vi "Image & ROI Update(SubVI).vi"(5 "Nr of Objects":dbl, 8 "error in (no error)":errorcluster, 9 "Numeric":dbl=50.0 format="%#_13g", 10 "Optical Flow Previous Image":T1, 11 "Refnum in":T1) -> (0 "error out":errorcluster, 1 "Rectangle":cluster{dbl, dbl, dbl, dbl, dbl}, 2 "ROI Descriptor":T2 {"Contours"."Type" items=["No Selection", "Point", "Line", "Rectangle", "Oval", "Polygon", "Freehand Region", "Annulus", "Unused2", "Unused3", "Broken Line", "Freehand Line", "Rotated Rectangle"]}, 3 "Refnum out":T1)   [LabVIEW 2014]
uses:
  <vilib>/vision/Image Controls.llb/IMAQ Image.ctl
  Global.vi
  <vilib>/vision/NI_Vision_Development_Module.lvlib
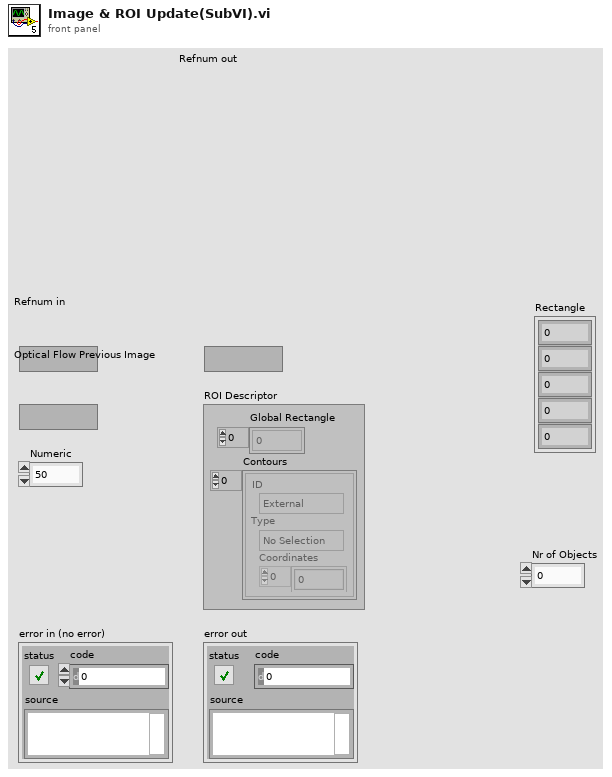
[diagram p1: front panel]
types:
  T1 = typedef "IMAQ Image.ctl" = refnum<image>
  T2 = typedef "ROI Descriptor" = cluster{"Global Rectangle":i32[], "Contours":cluster{"ID":enum32{"External", "Internal"}, "Type":u32, "Coordinates":i32[]}[]}
  T3 = typedef "Image Type" = u32
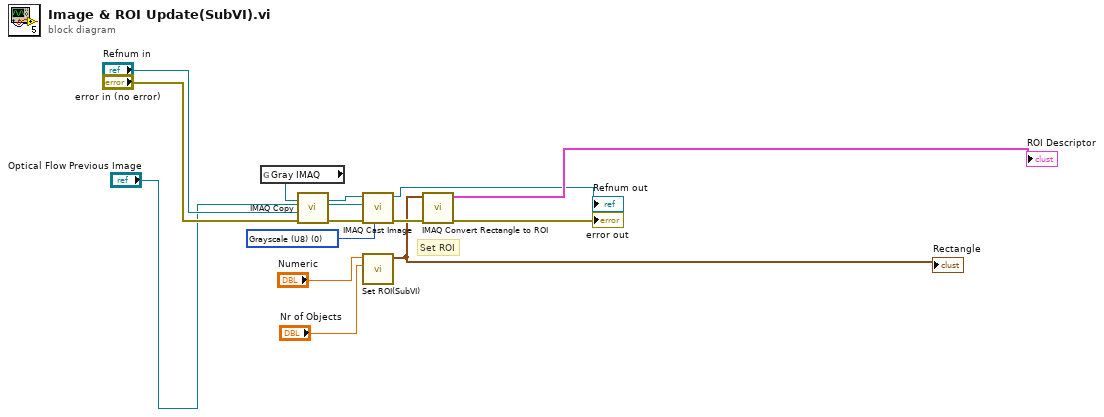
[diagram p0: block diagram]
diagram:
  w4 = T3 0 items=["Grayscale (U8)", "Grayscale (I16)", "Grayscale (SGL)", "Complex (CSG)", "RGB (U32)", "HSL (U32)", "RGB (U64)", "Grayscale (U16)"] ("Image Type")
  # "Set ROI"
  n1 = global read "Global.vi" "Gray IMAQ"() -> (w11:T1)
  n2 = call "IMAQ Copy"("error in (no error)"="error in (no error)", "Image Dst"="Refnum in", "Image Src"=w11) -> ("error out"=w10:errorcluster, "Image Dst Out"=w9:T1)  [unwired: 3 in]
  n3 = call "IMAQ Cast Image"("Image Type"=w4, "error in (no error)"=w10, "Image Dst"="Optical Flow Previous Image", "Image Src"=w9) -> ("error out"=w13:errorcluster, "Image Dst Out"=→"Refnum out":T1)  [unwired: 6 in]
  n4 = call "Set ROI(SubVI).vi"("Nr of objects"="Nr of Objects", "Numeric"="Numeric") -> ("Cluster"=w2:cluster{dbl, dbl, dbl, dbl, dbl})  [unwired: 9 in]
  "Rectangle" <- w2
  n5 = call "IMAQ Convert Rectangle to ROI"("error in (no error)"=w13, "Rectangle"=w2) -> ("error out"=→"error out":errorcluster, "ROI Descriptor"=→"ROI Descriptor":T2)  [unwired: 7 in]
